vi "DHE_SaveImgparams.vi"(4 "prefix":string="LASTIMG", 5 "sufix":string="LASTIMG", 6 "froot":string="LASTIMG", 7 "number":i32, 9 "basename":string="LASTIMG", 10 "dir":string="LASTIMG") -> ()   [LabVIEW 2016]
uses:
  <vilib>/Utility/config.llb/Write Key (String).vi
  <vilib>/Utility/config.llb/Write Key (I32).vi
  <vilib>/Utility/config.llb/NI_LVConfig.lvlib
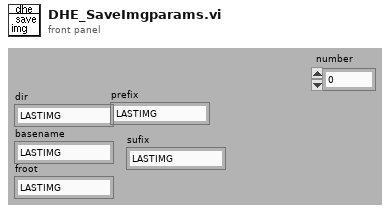
[diagram p1: front panel]
types:
  T1 = typedef "NI_LVConfig.lvlib/Config Data RefNum.ctl" = refnum<k1>
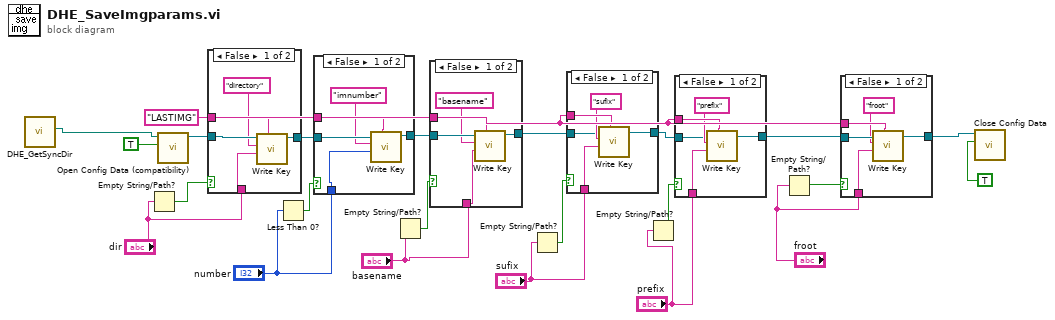
[diagram p0: block diagram]
diagram:
  w6 = "LASTIMG" ("section")
  n1 = call "DHE_GetSyncDir.vi"() -> ("sync file"=w1:path)  [unwired: 11 out]
  n2 = Empty String/Path?(string/path="dir") -> (empty?=w10:bool)
  n3 = call <vilib>:"Open Config Data (compatibility).vi"("create file if necessary (T)"=TRUE ("create file if necessary? (T)"), "configuration file path"=w1) -> ("refnum"=w23:T1)  [unwired: 7 in, 2 out]
  n4 = case shown="False" w10 {
    tunnel: w23 -> [w28 w29]
    tunnel: [w27 w29] -> w22
    tunnel: w6 -> [w25 _]
    tunnel: "dir" -> [w24 _]
    frame False {
      n5 = call-poly <vilib>:"Write Key.vi"("section"=w25, "value"=w24, "key"="directory", "refnum"=w28) -> ("refnum out"=w27:T1)  [unwired: 2 in, 5 out]
    }
    frame True {
    }
  }
  n6 = Less Than 0?(x="number") -> (x < 0?=w12:bool)
  n7 = case shown="False" w12 {
    tunnel: w22 -> [w34 w35]
    tunnel: [w33 w35] -> w19
    tunnel: w6 -> [w31 _]
    tunnel: "number" -> [w30 _]
    frame False {
      n8 = call-poly <vilib>:"Write Key.vi"("section"=w31, "value"=w30, "key"="imnumber", "refnum"=w34) -> ("refnum out"=w33:T1)  [unwired: 1 in, 6 out]
    }
    frame True {
    }
  }
  n9 = Empty String/Path?(string/path="basename") -> (empty?=w15:bool)
  n10 = case shown="False" w15 {
    tunnel: w19 -> [w40 w41]
    tunnel: [w38 w41] -> w3
    tunnel: w6 -> [w37 _]
    tunnel: "basename" -> [w36 _]
    frame False {
      n11 = call-poly <vilib>:"Write Key.vi"("section"=w37, "value"=w36, "key"="basename", "refnum"=w40) -> ("refnum out"=w38:T1)  [unwired: 2 in, 5 out]
    }
    frame True {
    }
  }
  n12 = Empty String/Path?(string/path="sufix") -> (empty?=w4:bool)
  n13 = case shown="False" w4 {
    tunnel: [w46 w47] -> w2
    tunnel: w3 -> [w42 w47]
    tunnel: w6 -> [w45 _]
    tunnel: "sufix" -> [w43 _]
    frame False {
      n14 = call-poly <vilib>:"Write Key.vi"("section"=w45, "value"=w43, "key"="sufix", "refnum"=w42) -> ("refnum out"=w46:T1)  [unwired: 2 in, 5 out]
    }
    frame True {
    }
  }
  n15 = Empty String/Path?(string/path="prefix") -> (empty?=w8:bool)
  n16 = case shown="False" w8 {
    tunnel: [w52 w53] -> w7
    tunnel: w2 -> [w48 w53]
    tunnel: w6 -> [w51 _]
    tunnel: "prefix" -> [w49 _]
    frame False {
      n17 = call-poly <vilib>:"Write Key.vi"("section"=w51, "value"=w49, "key"="prefix", "refnum"=w48) -> ("refnum out"=w52:T1)  [unwired: 2 in, 5 out]
    }
    frame True {
    }
  }
  n18 = Empty String/Path?(string/path="froot") -> (empty?=w16:bool)
  n19 = case shown="False" w16 {
    tunnel: [w58 w59] -> w18
    tunnel: w7 -> [w57 w59]
    tunnel: w6 -> [w56 _]
    tunnel: "froot" -> [w54 _]
    frame False {
      n20 = call-poly <vilib>:"Write Key.vi"("section"=w56, "value"=w54, "key"="froot", "refnum"=w57) -> ("refnum out"=w58:T1)  [unwired: 2 in, 5 out]
    }
    frame True {
    }
  }
  n21 = call <vilib>:"Close Config Data.vi"("write file if changed (T)"=TRUE ("write configuration file? (F)"), "refnum"=w18) -> ()  [unwired: 1 in, 9 out]
